vi "PH_BL-Master.get Boolean Status Service Subscriber Status by Name.vi"(0 "i ref in":refnum<vi>, 2 "Status Subscriber Instance":string="N/A", 5 "error in (no error)":errorcluster) -> (8 "Boolean GUI Ref":refnum<vi>, 9 "index of element":i32, 11 "no Link?":bool, 13 "Instance found?":bool, 14 "i ref out":refnum<vi>, 15 "off/false/out?":bool, 16 "on/true/in?":bool, 17 "Subscriber State":T1 items=["no info", "off/false/out", "on/true/in", "Failure", "Alarm", "Status 1", "Status 2", "Status 3"], 18 "off/false/out or on/true/in?":bool, 19 "error out":errorcluster)   [LabVIEW 2014, in "PH_BL-Master.lvlib"]
doc: "This VI gets the status of the selected Subscriber."
uses:
  PH_BL-Master.lvlib
  PH_StatusHandler/PH_StatusHandler.Status.ctl
  PH_StatusHandler/PH_StatusHandler.lvlib
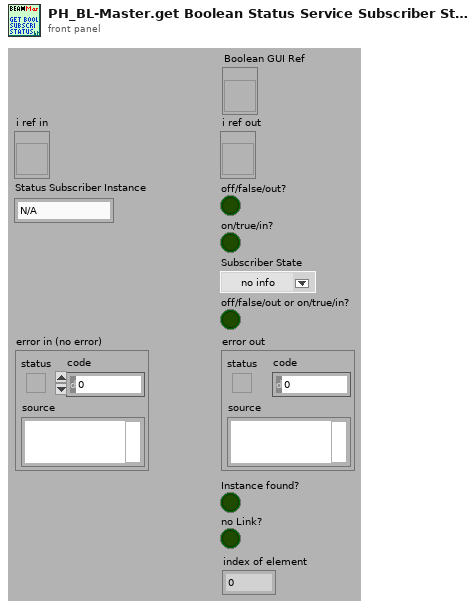
[diagram p1: front panel]
types:
  T1 = typedef "PH_StatusHandler.lvlib/PH_StatusHandler.Status.ctl" = i16
  T2 = typedef "PH_BL-Master.lvlib/PH_BL-Master.i attribute.ctl" = cluster{"Remote controlled":bool, "Boolean Condition Service Subscriber":refnum<vi>[], "Picture Condition Service Subscriber":refnum<vi>[], "R2S":cluster{"GUI Ref":refnum<vi>, "State":bool}, "Vacua":cluster{"GUI Ref":refnum<vi>, "Limit":dbl, "Curr Value":dbl, "in range":bool}[], "O2 Inspection":cluster{"GUI Ref":refnum<vi>, "Concentration":dbl, "State":T1}[], "Boolean Status Service Subscriber":cluster{"GUI Ref":refnum<vi>, "Status":T1, "no Link?":bool, "Status Subscriber Class":T3}[], "Picture Status Service Subscriber":cluster{"GUI Ref":refnum<vi>, "Status":T1, "no Link?":bool, "Status Subscriber Class":T3}[], "6P 4Q Service Subscriber":cluster{"GUI Ref":refnum<vi>, "Selector":T4, "no Link?":bool}[], "Index of latest 6P 4Q changing Instance":i32, "Index of latest Picture Status changing Instance":i32, "Index of latest Boolean Status changing Instance":i32, "Vision ID on same Node":string, "Start Phase over?":bool, "GUI Ref Delete":refnum<vi>}
  T3 = typedef "PH_BL-Master.lvlib/PH_BL-Master.Status Subscriber Class.ctl" = enum16{"unknown", "Switch", "BB", "6P Switch", "Switch GUI", "Switch and 6P State", "Force Sensor"}
  T4 = typedef "PH_4_Pos_Selector.lvlib/PH_4_Pos_Selector.Position Selector.ctl" = u16
  T5 = cluster{"GUI Ref":refnum<vi>, "Status":T1, "no Link?":bool, "Status Subscriber Class":T3}[]
  T6 = cluster{"GUI Ref":refnum<vi>, "Status":T1, "no Link?":bool, "Status Subscriber Class":T3}
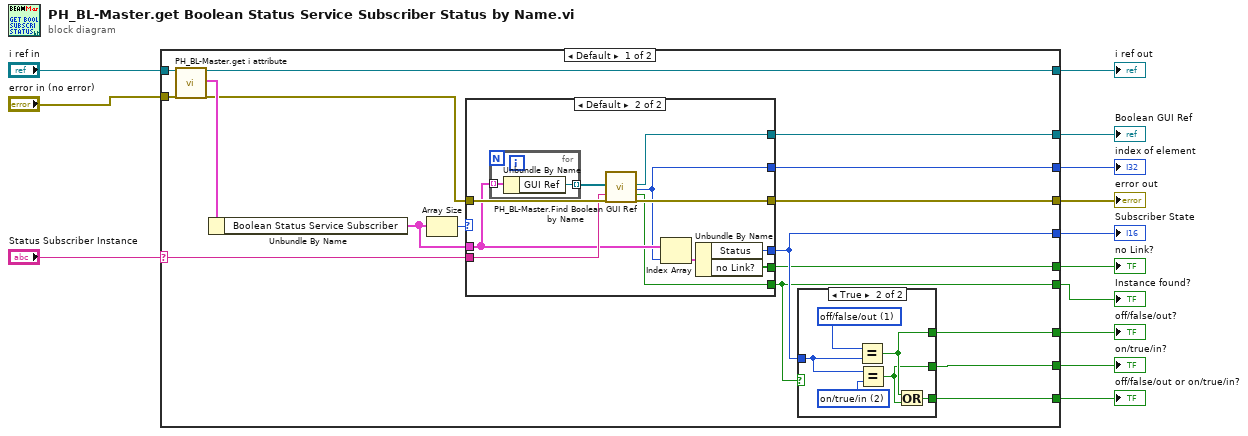
[diagram p0: block diagram]
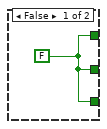
[diagram p2: hidden frame]
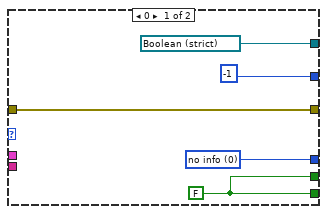
[diagram p3: hidden frame]
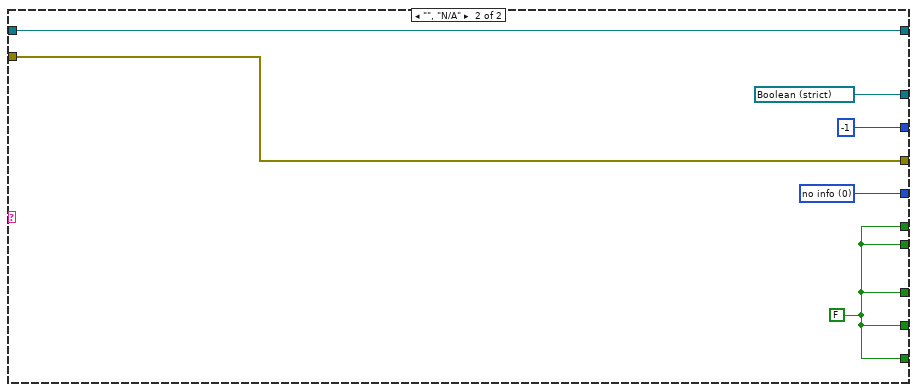
[diagram p4: hidden frame]
diagram:
  n1 = case shown="Default" "Status Subscriber Instance" {
    selector: "Status Subscriber Instance" -> [w23 _]
    tunnel: "error in (no error)" -> [w29 w60]
    tunnel: "i ref in" -> [w28 w61]
    tunnel: [w27 w61] -> w5
    tunnel: [w16 w59] -> w7
    tunnel: [w17 w60] -> w6
    tunnel: [w22 w57] -> w8
    tunnel: [w21 w57] -> w9
    tunnel: [w20 w57] -> w10
    tunnel: [w14 w57] -> w4
    tunnel: [w15 w57] -> w3
    tunnel: [w19 refnum<vi> refnum ("GUI Ref")] -> w2
    tunnel: [w18 -1 ("index of element")] -> w1
    frame Default {
      n2 = call "PH_BL-Master.get i attribute.vi"("i ref in"=w28, "error in (no error)"=w29) -> ("i ref out"=w27:refnum<vi>, "i attribute"=w30:T2, "error out"=w25:errorcluster)  [unwired: 15 in]
      n3 = Unbundle By Name(w30) -> ("Boolean Status Service Subscriber"=w24:T5)
      n4 = Array Size(array=w24) -> (size(s)=w26:i32)
      n5 = case shown="Default" w26 {
        tunnel: w24 -> [_ w48]
        tunnel: w23 -> [_ w51]
        tunnel: [w42 w49] -> w17
        tunnel: [w41 w45] -> w16
        tunnel: w25 -> [w42 w52]
        tunnel: [w39 w44] -> w14
        tunnel: [w39 w46] -> w15
        tunnel: [refnum<vi> refnum ("GUI Ref") w50] -> w19
        tunnel: [-1 ("index of element") w43] -> w18
        frame 0 {
          w39 = FALSE
          w41 = T1 0 items=["no info", "off/false/out", "on/true/in", "Failure", "Alarm", "Status 1", "Status 2", "Status 3"] ("State")
        }
        frame Default {
          n6 = for {
            tunnel: w48 -> [w55] mode=indexing
            tunnel: [w54] -> w53 mode=indexing
            n7 = Unbundle By Name(w55) -> ("GUI Ref"=w54:refnum<vi>)
          }
          n8 = call "PH_BL-Master.Find Boolean GUI Ref by Name.vi"("Boolean Ref Array"=w53, "Label"=w51, "error in (no error)"=w52) -> ("Wanted Boolean Ref"=w50:refnum<vi>, "index of element"=w43:i32, "Ref found?"=w44:bool, "error out"=w49:errorcluster)  [unwired: 13 in]
          n9 = Index Array(array=w48, index=w43) -> (element=w47:T6)
          n10 = Unbundle By Name(w47) -> ("Status"=w45:T1, "no Link?"=w46:bool)
        }
      }
      n11 = case shown="True" w14 {
        tunnel: [w31 w36] -> w22
        tunnel: [w31 w35] -> w21
        tunnel: [w31 w34] -> w20
        tunnel: w16 -> [_ w32]
        frame False {
          w31 = FALSE
        }
        frame True {
          w37 = T1 2 items=["no info", "off/false/out", "on/true/in", "Failure", "Alarm", "Status 1", "Status 2", "Status 3"] ("y")
          w33 = T1 1 items=["no info", "off/false/out", "on/true/in", "Failure", "Alarm", "Status 1", "Status 2", "Status 3"] ("y")
          n12 = Equal?(x=w33, y=w32) -> (x = y?=w36:bool)
          n13 = Equal?(x=w32, y=w37) -> (x = y?=w35:bool)
          n14 = Or(x=w36, y=w35) -> (x .or. y?=w34:bool)
        }
      }
    }
    frame "", "N/A" {
      w57 = FALSE
      w59 = T1 0 items=["no info", "off/false/out", "on/true/in", "Failure", "Alarm", "Status 1", "Status 2", "Status 3"] ("State")
    }
  }
  "i ref out" <- w5
  "error out" <- w6
  "Subscriber State" <- w7
  "off/false/out?" <- w8
  "on/true/in?" <- w9
  "off/false/out or on/true/in?" <- w10
  "Instance found?" <- w4
  "no Link?" <- w3
  "Boolean GUI Ref" <- w2
  "index of element" <- w1
